vi "Get_Sub_Collection.vi"(8 "error in (no error)":errorcluster caption="entrée d'erreur (pas d'erreur)", 11 "Firebase Altyor en entrée":refnum<class "Firebase Altyor.lvclass">) -> (0 "error out":errorcluster caption="sortie d'erreur", 3 "Firebase Altyor en sortie":refnum<class "Firebase Altyor.lvclass">)   [LabVIEW 2020, in "Library Instrument & Equipement.lvlib" / "Library FireBase.lvlib" / "Firebase Altyor.lvclass"]
doc: "Return the documents present in the test collection for each DATA read with Get_Data\nPlease initialise the following values\n - Name BDD\n - Document of test sequence\n - API Key\n - Nb To Read"
uses:
  Firebase Altyor.lvclass
  Firebase Altyor.lvclass/Firebase Altyor.ctl
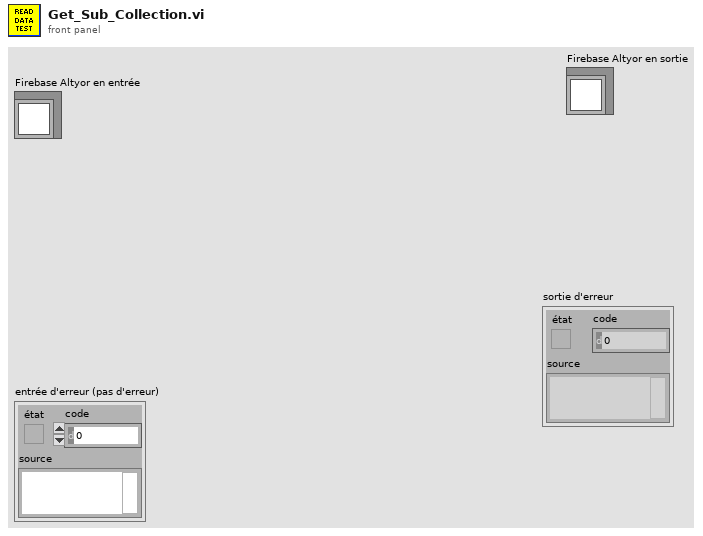
[diagram p1: front panel]
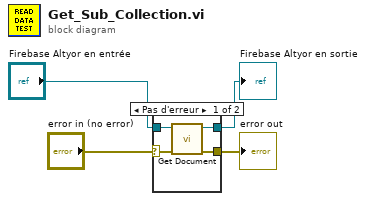
[diagram p0: block diagram]
diagram:
  n1 = case shown="Pas d'erreur" "error in (no error)" {
    selector: "error in (no error)" -> [w6 w10]
    tunnel: [w8 w10] -> w2
    tunnel: [w7 w9] -> w3
    tunnel: "Firebase Altyor en entrée" -> [w5 w9]
    frame No Error {
      n2 = call-dynamic "Get Document.vi"("error in (no error)"=w6, "Firebase (Default) en entrée"=w5) -> ("error out"=w8:errorcluster, "Firebase (Default) en sortie"=w7:refnum<class "Firebase Altyor.lvclass">)  [unwired: 8 in]
    }
    frame Error {
    }
  }
  "error out" <- w2
  "Firebase Altyor en sortie" <- w3
